vi "to_json.vi"(8 "error in":errorcluster, 11 "channelFilter in":refnum<class "channelFilter.lvclass">) -> (0 "error out":errorcluster, 2 "json":string, 3 "channelFilter out":refnum<class "channelFilter.lvclass">, 4 "Not Default":bool)   [LabVIEW 2020, in "nominal types.lvlib" / "channelFilter.lvlib" / "channelFilter.lvclass"]
uses:
  channelFilter.lvclass
  channelFilter.lvclass/channelFilter.ctl
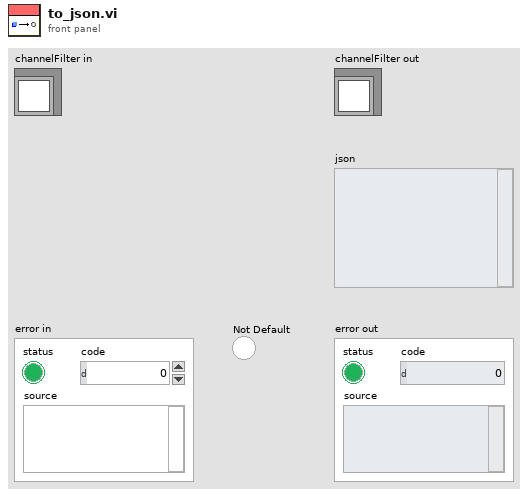
[diagram p1: front panel]
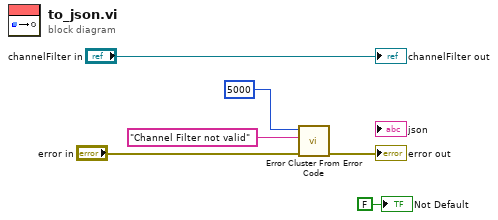
[diagram p0: block diagram]
diagram:
  n1 = call <vilib>:"Error Cluster From Error Code.vi"("error in (no error)"="error in", "error message (\"\")"="Channel Filter not valid" ("error message (\"\")"), "error code (0)"=5000) -> ("error out"=→"error out":errorcluster)  [unwired: 6 in]
  "channelFilter out" <- "channelFilter in"
  "Not Default" <- FALSE ("Not Default")
